vi "Get Class Path.vi"() -> ()   [LabVIEW 2014]
uses:
  reusable/General/Math/Fit Exponential Class/ExpFitLib.lvlibp/Children/LRS/LRS.lvclass
panel:
  out "class path":path
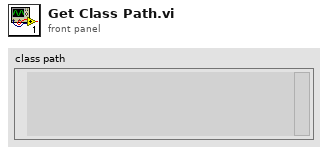
[diagram p1: front panel]
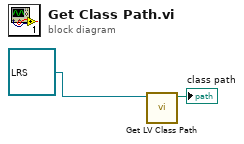
[diagram p0: block diagram]
diagram:
  n1 = call <vilib>:"Get LV Class Path.vi"("object"=refnum<class "LRS.lvclass"> refnum ("Exponential Fit Lib:LRS")) -> ("class path"=→"class path":path)  [unwired: 9 in, 1 out]
